vi "sendcmd.vi"(0 "VISA Refnum in":refnum<visa-resource-name>, 5 "write buffer":string, 11 "error in (no error)":errorcluster) -> (4 "VISA Refnum out":refnum<visa-resource-name>, 6 "read buffer":string, 15 "error out":errorcluster)   [LabVIEW 2020]
uses:
  haltnow.vi
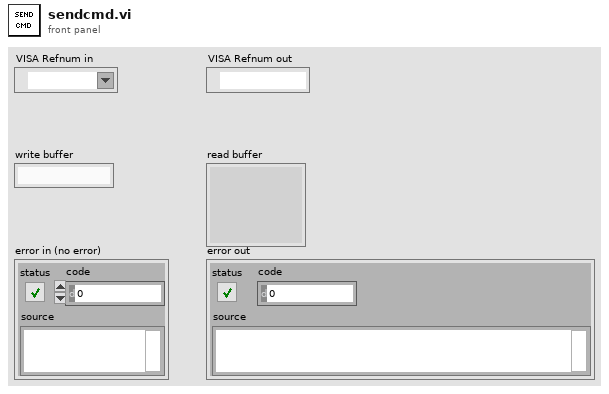
[diagram p1: front panel]
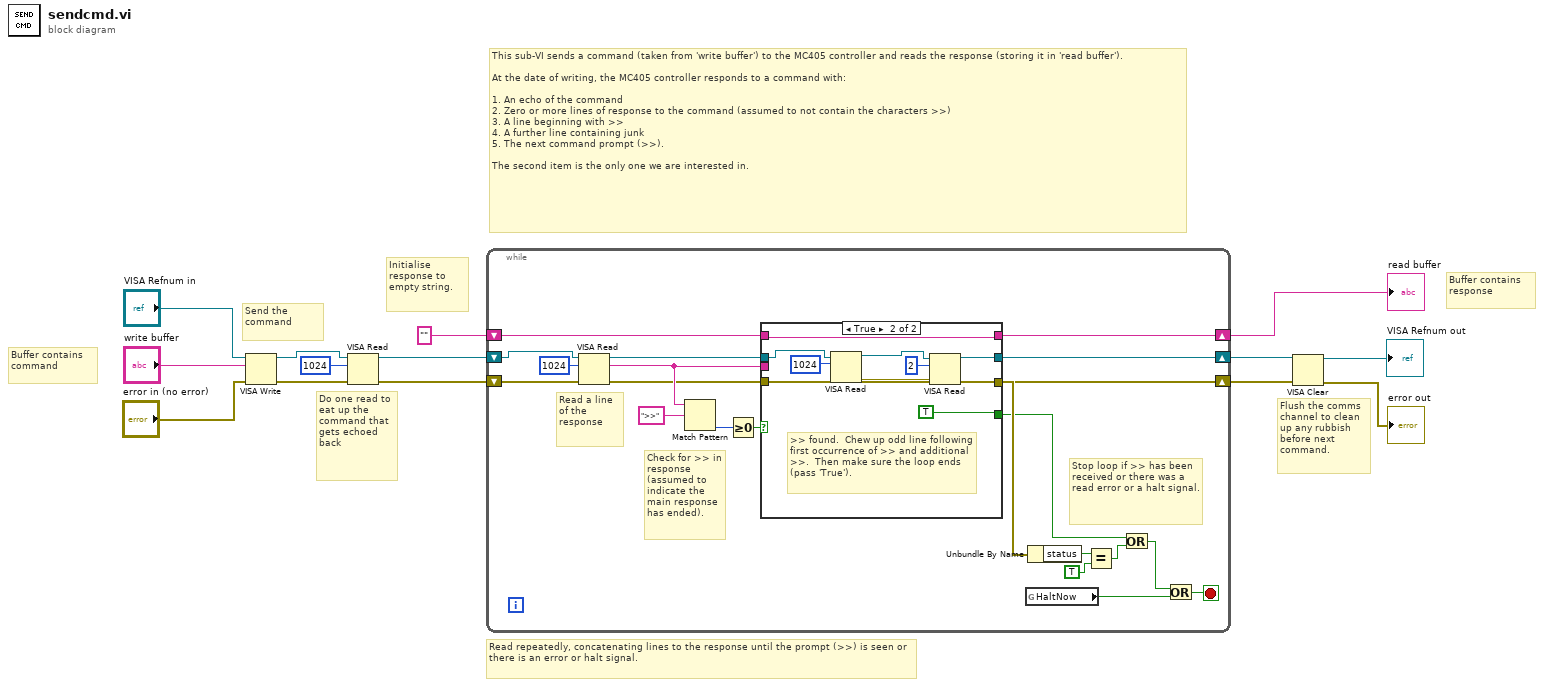
[diagram p0: block diagram]
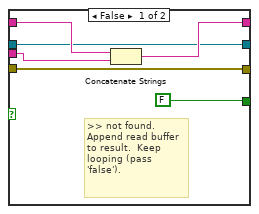
[diagram p2: hidden frame]
diagram:
  # "Send the command"
  # "Read repeatedly, concatenating lines to the response until the prompt (>>) is seen or there is an error or halt signal."
  # "Buffer contains command"
  # "This sub-VI sends a command (taken from 'write buffer') to the MC405 controller and reads the response (storing it in 'read buffer').\n\nAt the date of writing, the MC405 controller responds to a command with:\n\n1. An echo of the command \n2. Zero or more lines of response to the command (assumed to not contain the characters >>)\n3. A line beginning with >>\n4. A further line containing junk\n5. The next command prompt (>>).\n\nThe second item is the only one we are interested in."
  # "Buffer contains response"
  # "Initialise response to empty string."
  # "Flush the comms channel to clean up any rubbish before next command."
  # "Do one read to eat up the command that gets echoed back"
  n1 = VISA Write(VISA resource name="VISA Refnum in", write buffer="write buffer", error in (no error)="error in (no error)") -> (VISA resource name out=w10:refnum<visa-resource-name>, error out=w8:errorcluster)  [unwired: 1 out]
  n2 = VISA Read(VISA resource name=w10, byte count=u32 1024, error in (no error)=w8) -> (VISA resource name out=w9:refnum<visa-resource-name>, error out=w7:errorcluster)  [unwired: 2 out]
  n3 = while {
    shift-right: [w20] -> w2
    shift-left: w7 -> [w34]
    shift-right: [w19] -> w4
    shift-left: w9 -> [w33]
    shift-right: [w28] -> w12
    shift-left: "" -> [w29]
    stop <- w23 stop-if-true
    # "Stop loop if >> has been received or there was a read error or a halt signal."
    # "Read a line of the response"
    # "Check for >> in response (assumed to indicate the main response has ended)."
    n4 = VISA Read(VISA resource name=w33, byte count=u32 1024, error in (no error)=w34) -> (VISA resource name out=w22:refnum<visa-resource-name>, read buffer=w30:string, error out=w21:errorcluster)  [unwired: 1 out]
    n5 = Match Pattern(string=w30, regular expression=">>" ("y")) -> (offset past match=w18:i32)  [unwired: 1 in, 3 out]
    n6 = Greater Or Equal To 0?(x=w18) -> (x >= 0?=w31:bool)
    n7 = case shown="True" w31 {
      tunnel: w30 -> [w40 _]
      tunnel: w29 -> [w39 w41]
      tunnel: [w38 w41] -> w28
      tunnel: [FALSE TRUE] -> w16
      tunnel: w22 -> [w36 w49]
      tunnel: w21 -> [w35 w48]
      tunnel: [w35 w42] -> w20
      tunnel: [w36 w44] -> w19
      frame False {
        # ">> not found.  Append read buffer to result.  Keep looping (pass 'false')."
        n8 = Concatenate Strings(w39, w40) -> (w38:string)
      }
      frame True {
        # ">> found.  Chew up odd line following first occurrence of >> and additional >>.  Then make sure the loop ends (pass 'True')."
        n9 = VISA Read(VISA resource name=w49, byte count=u32 1024, error in (no error)=w48) -> (VISA resource name out=w45:refnum<visa-resource-name>, error out=w43:errorcluster)  [unwired: 2 out]
        n10 = VISA Read(VISA resource name=w45, byte count=u32 2, error in (no error)=w43) -> (VISA resource name out=w44:refnum<visa-resource-name>, error out=w42:errorcluster)  [unwired: 2 out]
      }
    }
    n11 = global read "haltnow.vi" "HaltNow"() -> (w25:bool)
    n12 = Unbundle By Name(w21) -> ("status"=w27:bool)
    n13 = Equal?(x=w27, y=TRUE) -> (x = y?=w17:bool)
    n14 = Or(x=w16, y=w17) -> (x .or. y?=w24:bool)
    n15 = Or(x=w24, y=w25) -> (x .or. y?=w23:bool)
  }
  "read buffer" <- w12
  n16 = VISA Clear(VISA resource name=w4, error in (no error)=w2) -> (VISA resource name out=→"VISA Refnum out":refnum<visa-resource-name>, error out=→"error out":errorcluster)
